vi "MDML_publish_data.vi"(0 "connMeta 4":T1, 1 "Data":string[](array[string]), 2 "Device ID":string, 3 "error in (no error)":errorcluster, 4 "Experiment ID":string) -> (6 "error out":errorcluster)   [LabVIEW 2018]
uses:
  Downloads/mqtt_lv2013_201708181938/mqtt_lv2013/mqtt Folder/src/class/mqtt/mqttTypedef/mqttConnectionMeta.ctl
  Downloads/mqtt_lv2013_201708181938/mqtt_lv2013/mqtt Folder/src/class/mqtt/mqttTypedef/mqttQOSlevel.ctl
  data_message.ctl
  Downloads/mqtt_lv2013_201708181938/mqtt_lv2013/mqtt Folder/src/class/mqtt/mqtt.lvclass
panel:
  out "MDML publish data errors":errorcluster
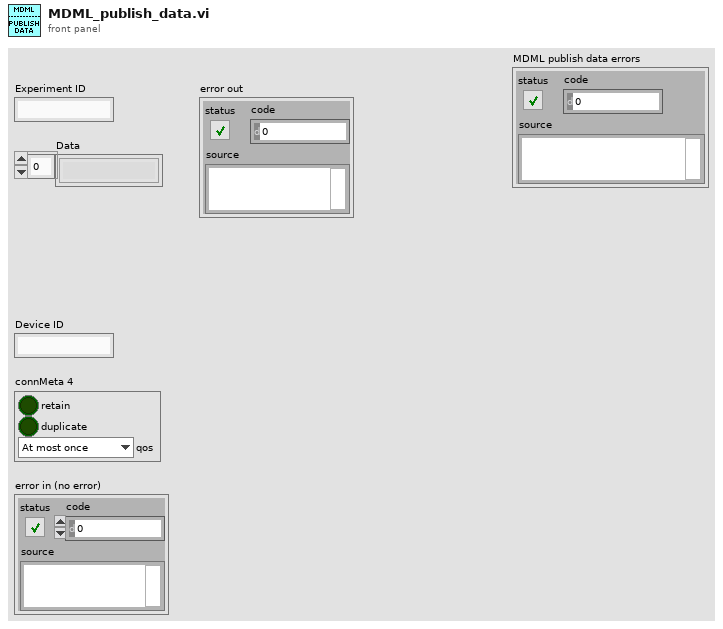
[diagram p1: front panel]
types:
  T1 = typedef "mqttConnectionMeta.ctl" = cluster{"retain":bool, "duplicate":bool, "qos":T2}
  T2 = typedef "mqttQOSlevel.ctl" = enum8{"At most once", "At least once", "Exactly once", "Reserved"}
  T3 = typedef "data_message.ctl" = cluster{"data":string, "data_delimiter":string, "influx_measurement":string}
  T4 = enum16{"Native", "Native Command Line", "UNIX", "Macintosh", "DOS"}
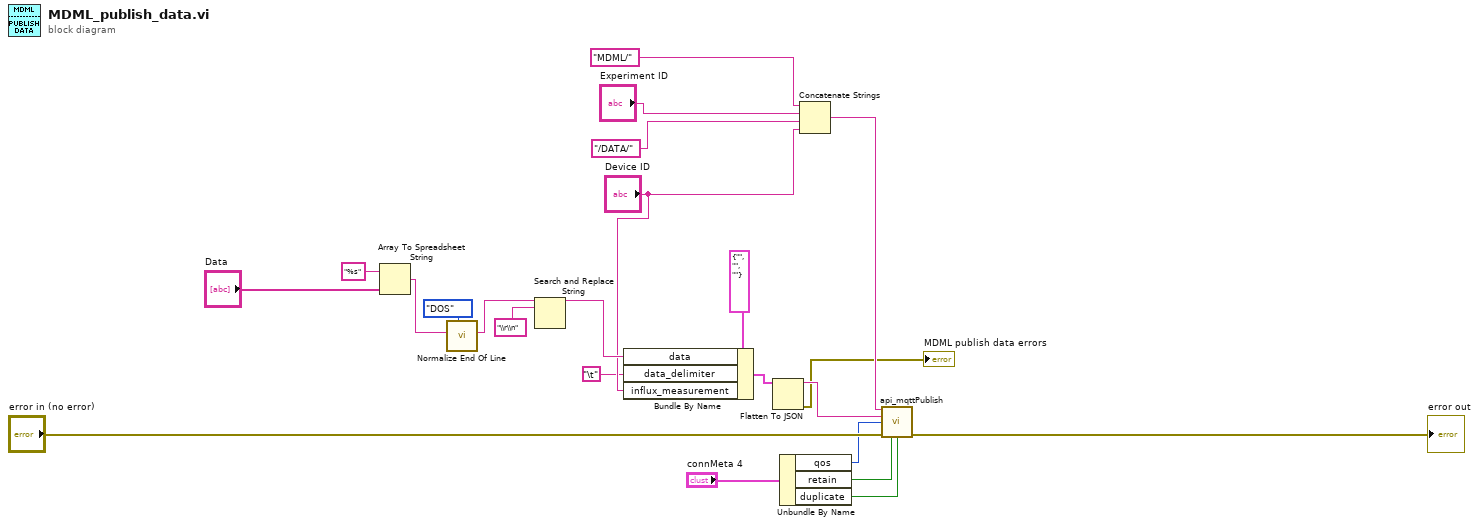
[diagram p0: block diagram]
diagram:
  n1 = Array To Spreadsheet String(array="Data", 3:"%s" ("format string")) -> (spreadsheet string=w17:string)  [unwired: 1 in]
  n2 = call <vilib>:"Normalize End Of Line.vi"("end of line (Native)"=T4."DOS", "string in"=w17) -> ("string out"=w19:string)  [unwired: 6 in]
  n3 = Search and Replace String(input string=w19, search string="\\r\\n") -> (result string=w20:string)  [unwired: 6 in, 3 out]
  n4 = Bundle By Name(cluster=T3 {"data"="", "data_delimiter"="", "influx_measurement"=""} ("input cluster"), "data"=w20, "data_delimiter"="\t", "influx_measurement"="Device ID") -> (w22:T3)
  n5 = Flatten To JSON(anything=w22) -> (JSON string=w23:string, 11:→"MDML publish data errors":errorcluster)  [unwired: 2 in]
  n6 = Unbundle By Name("connMeta 4") -> ("qos"=w10:T2, "retain"=w11:bool, "duplicate"=w12:bool)
  n7 = Concatenate Strings("MDML/", "Experiment ID", "/DATA/", "Device ID") -> (w3:string)
  n8 = call "api_mqttPublish.vi"("topic"=w3, "value"=w23, "QoS (At most once)"=w10, "error in (no error)"="error in (no error)", "retain(F)"=w11, "duplicate(F)"=w12) -> ("error out"=→"error out":errorcluster)  [unwired: 8 in, 1 out]
